vi "3-11.vi"() -> ()   [LabVIEW 2022 SP3]
panel:
  out "数组":dbl[](array[numeric])
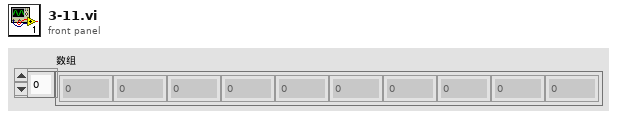
[diagram p1: front panel]
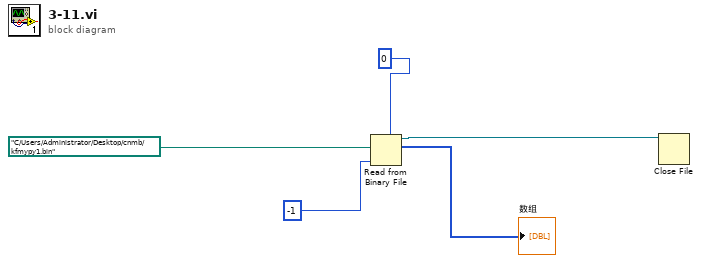
[diagram p0: block diagram]
diagram:
  n1 = Read from Binary File(5:0, 10:-1 ("计数"), 11:path "C:/Users/Administrator/Desktop/cnmb/kfmypy1.bin" ("文件（使用对话框）")) -> (2:→"数组":i32[], 3:w2:refnum<file>)  [unwired: 3 in, 2 out]
  n2 = Close File(refnum=w2) -> ()  [unwired: 1 in, 2 out]
